vi "Read UI Info From Configuration.vi"(8 "error in (no error)":errorcluster, 11 "node in":refnum<class "RIO Target.lvclass">) -> (0 "error out":errorcluster, 1 "Destination Path":path, 2 "VI to Place Engines and IO Nodes":path, 3 "node out":refnum<class "RIO Target.lvclass">, 5 "Target Project Path":path)   [LabVIEW 2014, in "RIO Target.lvclass"]
uses:
  RIO Target.lvclass
  RIO Target.lvclass/RIO Target.ctl
  <vilib>/NI/Configuration Framework/serializable configuration/read metadata property.vi
  RIO Target Configuration/RIO Target Configuration.lvclass
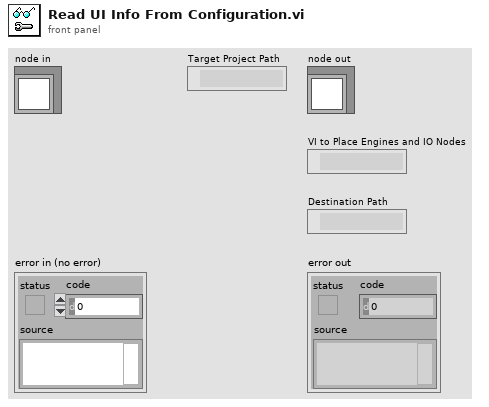
[diagram p1: front panel]
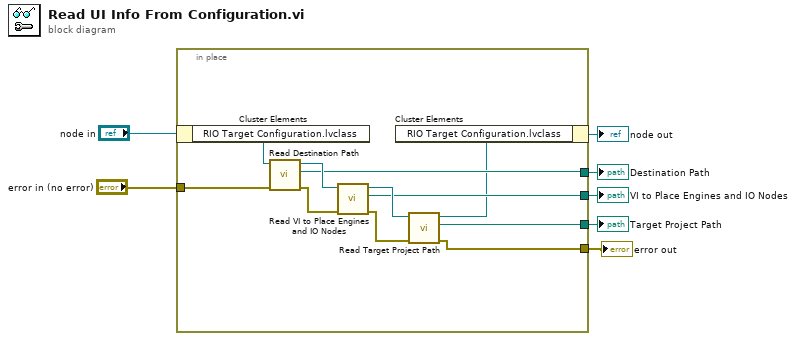
[diagram p0: block diagram]
diagram:
  n1 = in-place {
    in-place-border: [w15] -> w6
    in-place-border: [w14] -> w5
    in-place-border: [w13] -> w4
    in-place-border: "error in (no error)" -> [w12]
    in-place-border: [w8] -> w1
    n2 = in-place-cluster #1("node in") -> ("RIO Target Configuration.lvclass"=w18:refnum<class "RIO Target Configuration.lvclass">)
    n3 = call "Read Destination Path.vi"("error in (no error)"=w12, "RIO Target Configuration in"=w18) -> ("error out"=w11:errorcluster, "Destination Path"=w15:path, "RIO Target Configuration out"=w17:refnum<class "RIO Target Configuration.lvclass">)  [unwired: 7 in]
    n4 = call "Read VI to Place Engines and IO Nodes.vi"("error in (no error)"=w11, "RIO Target Configuration in"=w17) -> ("error out"=w10:errorcluster, "VI to Place Engines and IO Nodes"=w14:path, "RIO Target Configuration out"=w16:refnum<class "RIO Target Configuration.lvclass">)  [unwired: 7 in]
    n5 = call "Read Target Project Path.vi"("error in (no error)"=w10, "RIO Target Configuration in"=w16) -> ("error out"=w8:errorcluster, "Target Project Path"=w13:path, "RIO Target Configuration out"=w9:refnum<class "RIO Target Configuration.lvclass">)  [unwired: 7 in]
    n6 = in-place-cluster #1("RIO Target Configuration.lvclass"=w9) -> (→"node out":refnum<class "RIO Target.lvclass">)
  }
  "Destination Path" <- w6
  "VI to Place Engines and IO Nodes" <- w5
  "Target Project Path" <- w4
  "error out" <- w1
